vi "Configure Frequency Gate.vi"(6 "Measurement Mode (0: Auto)":i32(ring) items=["Auto", "Reciprocal", "Continuous"], 7 "Polarity (1: Negative)":i32(ring)=1 items=["Positive", "Negative"], 8 "error in (no error)":errorcluster, 9 "Time Resolution (0.1 s)":dbl=0.1, 10 "Gate Source (0: Time)":i32(ring) items=["Time", "External", "Input1", "Input2", "Advanced"], 11 "VISA resource name":refnum<visa-resource-name>) -> (0 "error out":errorcluster, 3 "VISA resource name out":refnum<visa-resource-name>)   [LabVIEW 2024, in "Agilent 532XX Series.lvlib"]
doc: "Configures the characteristics of frequency gate."
uses:
  Agilent 532XX Series.lvlib
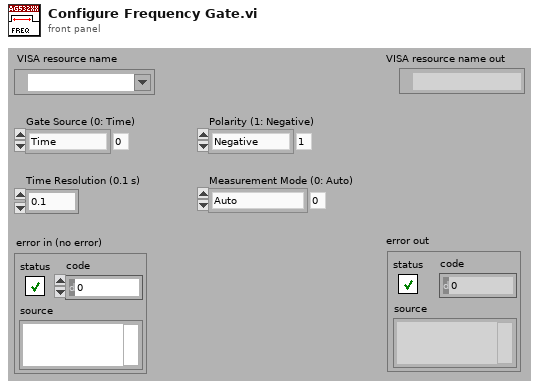
[diagram p1: front panel]
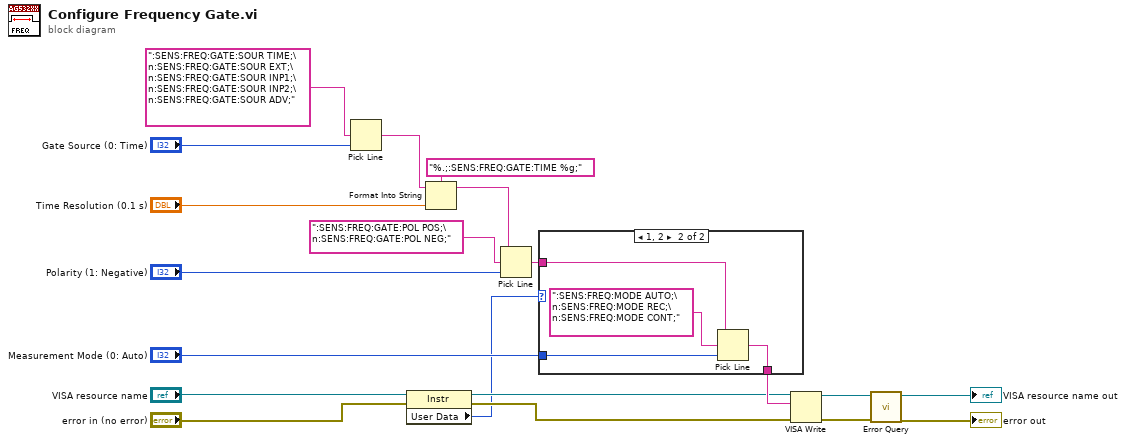
[diagram p0: block diagram]
diagram:
  n1 = Pick Line(multi-line string=":SENS:FREQ:GATE:SOUR TIME;\n:SENS:FREQ:GATE:SOUR EXT;\n:SENS:FREQ:GATE:SOUR INP1;\n:SENS:FREQ:GATE:SOUR INP2;\n:SENS:FREQ:GATE:SOUR ADV;", line index="Gate Source (0: Time)") -> (output string=w18:string)  [unwired: 1 out]
  n2 = property class="Instr"(reference="VISA resource name", error in="error in (no error)") -> (reference out=w3:refnum<visa-resource-name>, error out=w4:errorcluster, "User Data"=w1:u32)
  n3 = Format Into String(format string="%.;:SENS:FREQ:GATE:TIME %g;", initial string=w18, "Time Resolution (0.1 s)") -> (resulting string=w13:string)  [unwired: 1 in, 1 out]
  n4 = Pick Line(string ("")=w13, multi-line string=":SENS:FREQ:GATE:POL POS;\n:SENS:FREQ:GATE:POL NEG;", line index="Polarity (1: Negative)") -> (output string=w11:string)
  n5 = case shown="1, 2" w1 {
    tunnel: "Measurement Mode (0: Auto)" -> [_ w24]
    tunnel: w11 -> [w21 w23]
    tunnel: [w21 w22] -> w10
    frame 0, Default {
    }
    frame 1, 2 {
      n6 = Pick Line(string ("")=w23, multi-line string=":SENS:FREQ:MODE AUTO;\n:SENS:FREQ:MODE REC;\n:SENS:FREQ:MODE CONT;", line index=w24) -> (output string=w22:string)
    }
  }
  n7 = VISA Write(VISA resource name=w3, write buffer=w10, error in (no error)=w4) -> (VISA resource name out=w9:refnum<visa-resource-name>, error out=w8:errorcluster)  [unwired: 1 out]
  n8 = call "Error Query.vi"("error in (no error)"=w8, "VISA resource name"=w9) -> ("error out"=→"error out":errorcluster, "VISA resource name out"=→"VISA resource name out":refnum<visa-resource-name>)  [unwired: 8 out]
